vi "Read From Spreadsheet File (string) errors.vi"(0 "file path (dialog if empty)":path, 2 "number of rows (all:-1)":i32=-1, 5 "start of read offset (chars.:0)":i32, 6 "max characters/row  (no limit:0)":i32, 7 "error in (not an error)":errorcluster, 10 "format (%s)":string="%s", 11 "transpose (no:F)":bool, 17 "delimiter (\\t)":string="\t") -> (16 "new file path (Not A Path if cancelled)":path, 20 "all rows":string[][](array[string]), 22 "first row":string[](array[string]), 25 "mark after read (chars.)":i32, 26 "EOF?":bool, 27 "error out":errorcluster)   [LabVIEW 2018, in "Test Number and Bin Generator.lvlib" / "Test Number and Bin Generator.lvclass"]
doc: "Reads a specified number of lines or rows from a numeric text file beginning at a specified character offset and converts the data to a 2D, double-precision array of numbers, strings, or integers. You must manually select the polymorphic instance you want to use."
uses:
  Test Number and Bin Generator.lvclass
panel:
  in  "type (empty)":string[][](array[string])
  # "row\ncolumn"
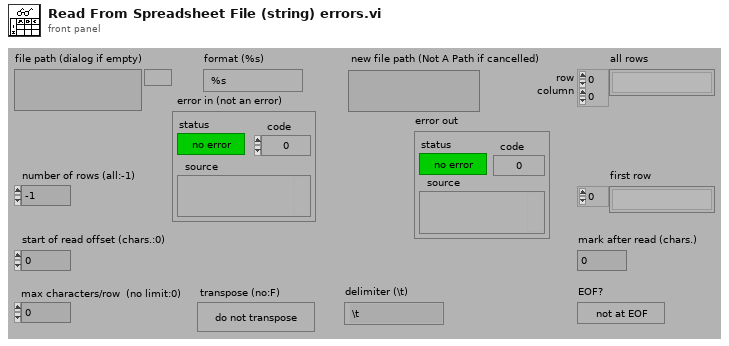
[diagram p1: front panel]
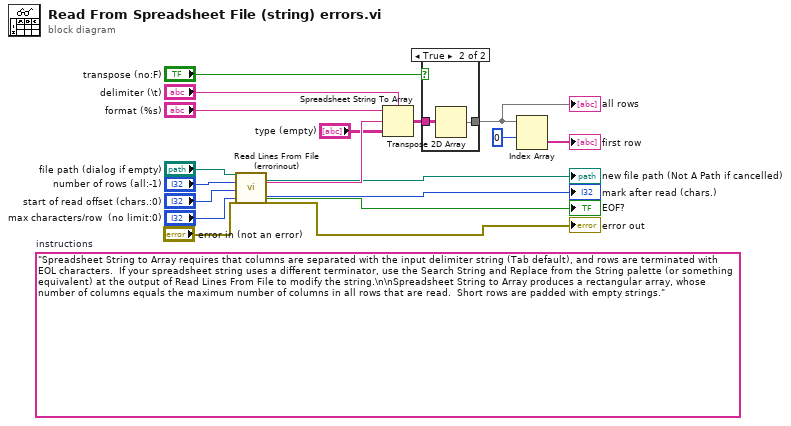
[diagram p0: block diagram]
diagram:
  (unwired) "Spreadsheet String to Array requires that columns are separated with the input delimiter string (Tab default), and rows are terminated with EOL characters.  If your spreadsheet string uses a different terminator, use the Search String and Replace from the String palette (or something equivalent) at the output of Read Lines From File to modify the string.\n\nSpreadsheet String to Array produces a rectangular array, whose number of columns equals the maximum number of columns in all rows that are read.  Short rows are padded with empty strings."  # instructions
  n1 = call "Read Lines From File (errorinout).vi"("file path (dialog if empty)"="file path (dialog if empty)", "number of lines (all:-1)"="number of rows (all:-1)", "start of read offset (chars.:0)"="start of read offset (chars.:0)", "[max characters per line]  (no limit:0)"="max characters/row  (no limit:0)", "error in (not an error)"="error in (not an error)") -> ("new file path (Not A Path if cancelled)"=→"new file path (Not A Path if cancelled)":path, "mark after read (chars.)"=→"mark after read (chars.)":i32, "line string"=w14:string, "EOF?"=→"EOF?":bool, "error out"=→"error out":errorcluster)  [unwired: 18 in]
  n2 = Spreadsheet String To Array(delimiter (Tab)="delimiter (\\t)", format string="format (%s)", spreadsheet string=w14, array type (2D Dbl)="type (empty)") -> (array=w5:string[][])
  n3 = case shown="True" "transpose (no:F)" {
    tunnel: w5 -> [w19 w21]
    tunnel: [w19 w20] -> w3
    frame False {
    }
    frame True {
      n4 = Transpose 2D Array(2D array=w21) -> (transposed array=w20:string[][])
    }
  }
  "all rows" <- w3
  n5 = Index Array(array=w3, index (row)=0) -> (element=→"first row":string[])  [unwired: 1 in]
